vi "Calib_Ref_info.vi"(1 "Input string":string, 2 "Reference Name":string="Instrument to calibrate") -> (0 "Reference instrument":T2={"high limit (10V)"=4.0, "low limit (-10V)"=0.0, "Ch No"=4, "Off ch no"=0, "Calib filename"=path "", "Ref Instrument type"=enum."Enter Value", "DAQmx Channel"=""} {"Off ch no" min=0 max=1; "Ch No" min=0 max=50; "low limit (-10V)" min=-10 max=10 format="%.1f"; "high limit (10V)" min=-10 max=10 format="%.1f"})   [LabVIEW 2013]
uses:
  Calib_setup.ctl
  Controls/Ref_Inst_type.ctl
panel:
  in  "Ref Instrument type":T1=enum."Generic Linear"
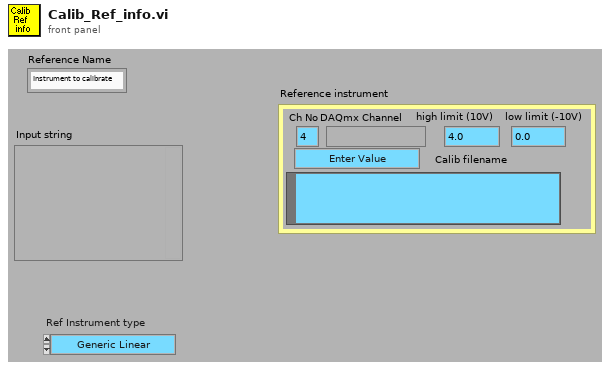
[diagram p1: front panel]
types:
  T1 = typedef "Ref_Inst_type.ctl" = enum16{"Propellor anemometer", "Pressure Transducer", "Raw voltage", "Pitot-static tube", "Preston tube", "Generic Linear", "Generic Polynomial", "Thermocouple", "LDA", "Enter Value", "ADAM Channel"}
  T2 = typedef "Calib_setup.ctl" = cluster{"high limit (10V)":sgl, "low limit (-10V)":sgl, "Ch No":i16, "Off ch no":i8, "Calib filename":path, "Ref Instrument type":T1, "DAQmx Channel":tag}
  T3 = cluster{"high limit (10V)":sgl, "low limit (-10V)":sgl, "Ch No":i16, "Off ch no":i8, "Calib filename":path, "Ref Instrument type":enum16{"Propellor anemometer", "Pressure Transducer", "Raw voltage", "Pitot-static tube", "Generic Inst", "Thermocouple", "LDA", "Enter Value", "ADAM Channel"}, "DAQmx Physical Channel":tag}
  T4 = enum16{"Propellor anemometer", "Pressure Transducer", "Raw voltage", "Pitot-static tube", "Generic Inst", "Thermocouple", "LDA", "Enter Value", "ADAM Channel"}
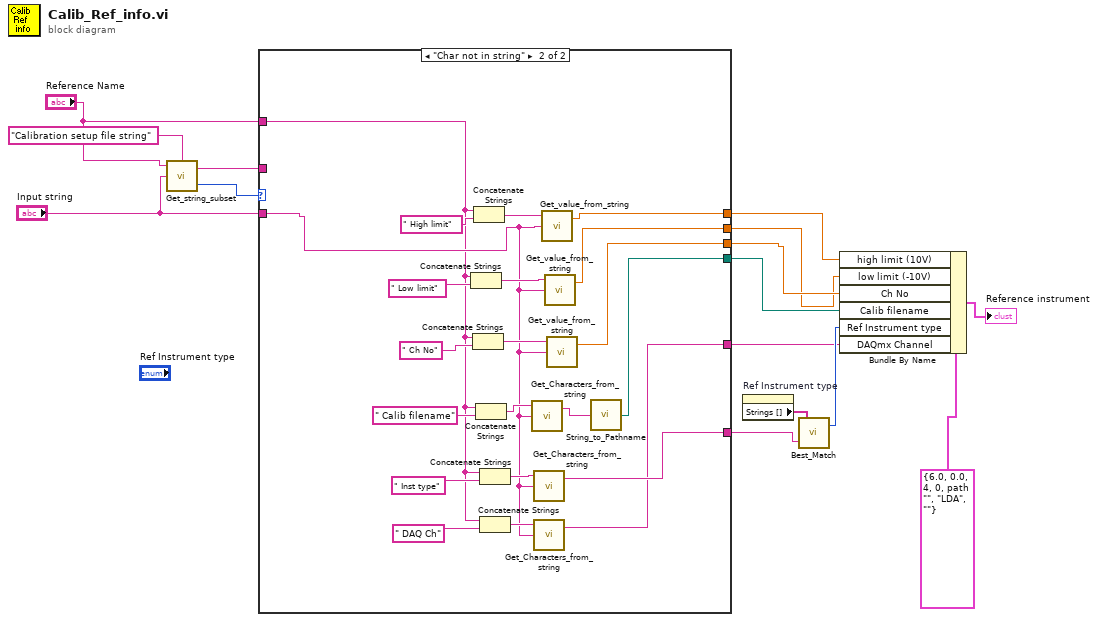
[diagram p0: block diagram]
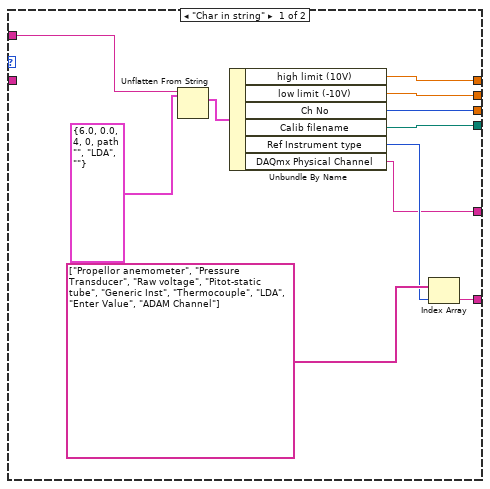
[diagram p2: hidden frame]
diagram:
  n1 = call "Get_string_subset.vi"("String Name"="Calibration setup file string", "String to split"="Input string", "File Label"="Reference Name") -> ("Status"=w14:enum16{"Char in string", "Char not in string"}, "Output string"=w13:string)  [unwired: 1 in]
  n2 = case shown="\"Char not in string\"" w14 {
    tunnel: "Input string" -> [_ w29]
    tunnel: w13 -> [w26 _]
    tunnel: "Reference Name" -> [_ w28]
    tunnel: [w21 w32] -> w8
    tunnel: [w20 w33] -> w6
    tunnel: [w19 w34] -> w5
    tunnel: [w18 w35] -> w4
    tunnel: [w17 w36] -> w3
    tunnel: [w16 w27] -> w1
    frame "Char in string" {
      n3 = Unflatten From String(type=T3 {"high limit (10V)"=6.0, "low limit (-10V)"=0.0, "Ch No"=4, "Off ch no"=0, "Calib filename"=path "", "Ref Instrument type"=enum."LDA", "DAQmx Physical Channel"=""} ("Ref vel for angle calib"), binary string=w26) -> (value=w24:T3)  [unwired: 1 in, 4 out]
      n4 = Unbundle By Name(w24) -> ("high limit (10V)"=w17:sgl, "low limit (-10V)"=w18:sgl, "Ch No"=w19:i16, "Calib filename"=w20:path, "Ref Instrument type"=w22:T4, "DAQmx Physical Channel"=w16:tag)
      n5 = Index Array(array=string[] ["Propellor anemometer", "Pressure Transducer", "Raw voltage", "Pitot-static tube", "Generic Inst", "Thermocouple", "LDA", "Enter Value", "ADAM Channel"] ("Strings []"), index=w22) -> (element=w21:string)
    }
    frame "Char not in string" {
      n6 = Concatenate Strings(w28, " Low limit") -> (w42:string)
      n7 = Concatenate Strings(w28, " Ch No") -> (w43:string)
      n8 = Concatenate Strings(w28, " High limit") -> (w44:string)
      n9 = Concatenate Strings(w28, " Calib filename") -> (w39:string)
      n10 = Concatenate Strings(w28, " Inst type") -> (w37:string)
      n11 = Concatenate Strings(w28, " DAQ Ch") -> (w30:string)
      n12 = call "Get_Characters_from_string.vi"("Input string"=w29, "Variable name"=w39) -> ("Value"=w38:string)  [unwired: 1 in, 1 out]
      n13 = call "Get_Characters_from_string.vi"("Input string"=w29, "Variable name"=w37) -> ("Value"=w32:string)  [unwired: 1 in, 1 out]
      n14 = call "Get_Characters_from_string.vi"("Input string"=w29, "Variable name"=w30) -> ("Value"=w27:string)  [unwired: 1 in, 1 out]
      n15 = call "Get_value_from_string.vi"("Input string"=w29, "Variable name"=w44) -> ("Value"=w36:dbl)  [unwired: 1 in, 1 out]
      n16 = call "Get_value_from_string.vi"("Input string"=w29, "Variable name"=w42) -> ("Value"=w35:dbl)  [unwired: 1 in, 1 out]
      n17 = call "Get_value_from_string.vi"("Input string"=w29, "Variable name"=w43) -> ("Value"=w34:dbl)  [unwired: 1 in, 1 out]
      n18 = call "String_to_Pathname.vi"("Input String"=w38) -> ("path"=w33:path)
    }
  }
  n19 = property on="Ref Instrument type" class="Enum (strict)"() -> ("Strings []"=w9:string[])  [unwired: 2 in, 2 out]
  n20 = call "Best_Match.vi"("Input String"=w8, "String Options"=w9) -> ("index of element"=w7:i32)  [unwired: 1 out]
  n21 = Bundle By Name(cluster=T2 {"high limit (10V)"=6.0, "low limit (-10V)"=0.0, "Ch No"=4, "Off ch no"=0, "Calib filename"=path "", "Ref Instrument type"=enum."LDA", "DAQmx Channel"=""} ("Reference instrument"), "high limit (10V)"=w3, "low limit (-10V)"=w4, "Ch No"=w5, "Calib filename"=w6, "Ref Instrument type"=w7, "DAQmx Channel"=w1) -> (→"Reference instrument":T2)
